vi "光源測試2.vi"() -> ()   [LabVIEW 2015]
uses:
  <vilib>/userdefined/High Color/IMAQdx.ctl
  Function/Control 5.ctl
  <vilib>/vision/Image Controls.llb/IMAQ Image.ctl
  <vilib>/vision/driver/NI_Vision_Acquisition_Software.lvlib
  <vilib>/vision/NI_Vision_Development_Module.lvlib
panel:
  in  "Action 15":bool
  in  "Action 14":bool
  in  "Action 13":bool
  in  "Action 12":bool
  in  "Action 11":bool
  out "Image 4":T1(plugin-control)
  out "error out 2":errorcluster
  out "# elements in queue":i32
  in  "Action 10":bool
  in  "Action 9":bool
  in  "Action 8(平均儲存)":bool
  in  "Action 7(キА)":bool
  in  "Action 6(清除)":bool
  out "Image 3":T1(plugin-control)
  out "Image 2":T1(plugin-control)
  out "Image 1":T1(plugin-control)
  out "Image 0":T1(plugin-control)
  out "Image":T1(plugin-control)
  out "Array":T1[](array[plugin-control])
  out "Numeric":i8 min=0 max=5 step=1
  out "Image_Array":T1[](array[typedef])
  in  "Image_Enum":T2(ring)
  in  "光源VISA":refnum<visa-resource-name>="COM14"
  out "element":T3
  in  "連續取像":bool
  in  "相機VISA":T4="cam14"
  in  "儲存影像":bool
  in  "觸發取像":bool
  in  "光源亮度 total":u8(slide) scale=0.0..255.0
  in  "milliseconds to wait":u32=200
  in  "Action 5(無)":bool
  in  "Action 4(拍照不存)":bool
  in  "Action 3(邊拍邊存)":bool
  in  "Action 2(全關)":bool
  in  "Action 1(全開)":bool
  out "回應值4":string
  out "回應值3":string
  out "回應值2":string
  out "回應值1":string
  in  "光源亮度 4":u8(slide) scale=0.0..255.0
  in  "光源亮度 3":u8(slide) scale=0.0..255.0
  in  "光源亮度 2":u8(slide) scale=0.0..255.0
  in  "光源亮度 1":u8(slide) scale=0.0..255.0
  in  "光源開啟 4":bool
  in  "光源開啟 3":bool
  in  "光源開啟 2":bool
  in  "光源開啟 1":bool
  in  "光源關閉 4":bool
  in  "光源關閉 3":bool
  in  "光源關閉 2":bool
  in  "通訊關閉":bool
  in  "光源關閉 1":bool
  in  "初始化":bool
  in  "Stop Button":bool
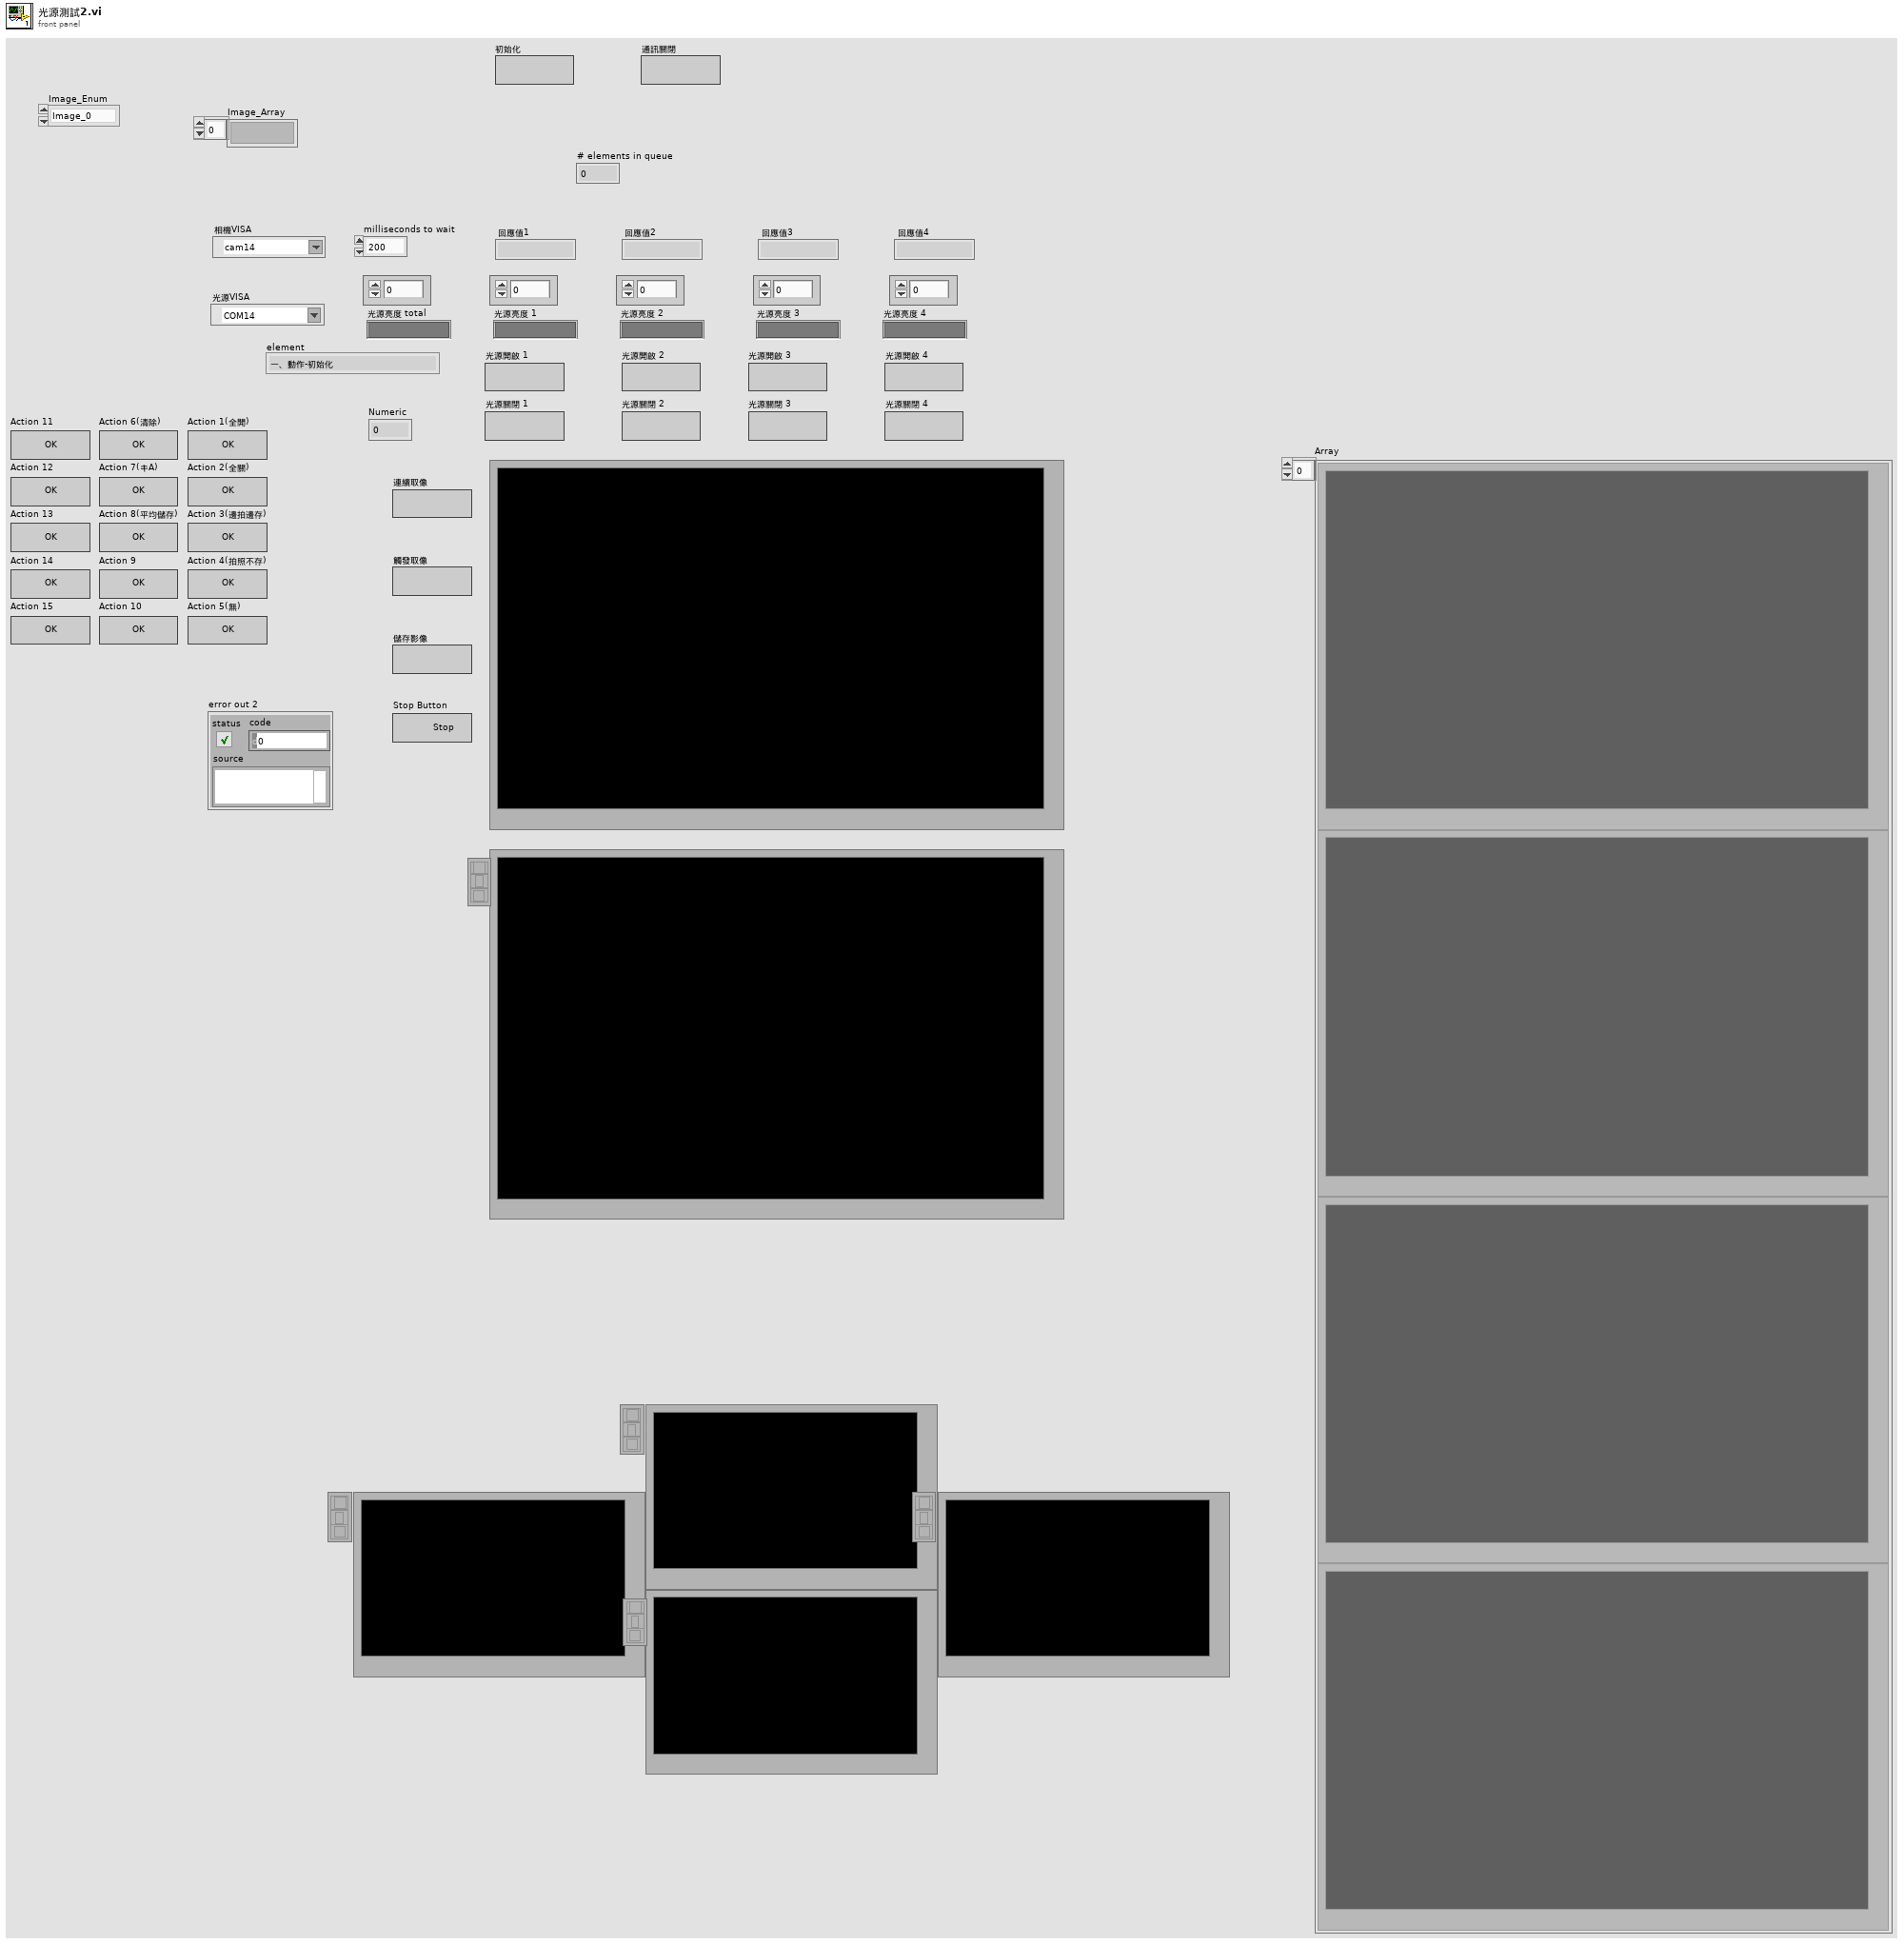
[diagram p1: front panel]
types:
  T1 = typedef "IMAQ Image.ctl" = refnum<image>
  T2 = enum16{"Image_0", "Image_1", "Image_2", "Image_3", "Image_4", "Image_5", "Image_6"}
  T3 = typedef "Control 5.ctl" = enum16{"一、動作-初始化", "二、動作-單次取像", "三、動作-連續取像", "四、動作-儲存影像", "五、動作-閒置", "六、動作-離開", "CH1_Open", "CH2_Open", "CH3_Open", "CH4_Open", "CH1_Close", "CH2_Close", "CH3_Close", "CH4_Close", "Action1", "Action2", "Action3", "Action4", "Action5", "Action6", "Action7", "Action8", "Action9", "Action10", "Action11", "Action12", "Action13", "Action14", "Action15"}
  T4 = typedef "IMAQdx.ctl" = refnum<k21>
  T5 = typedef "光源通訊_action_control.ctl" = enum16{"initial", "開啟光源", "關閉光源", "close"}
  T6 = typedef "Image Type" = u32
  T7 = typedef "LVDateTimeRec.ctl" = cluster{"fractional second":dbl, "second":i32, "minute":i32, "hour":i32, "day of month":i32, "month":i32, "year":i32, "day of week":i32, "day of year":i32, "DST":i32}
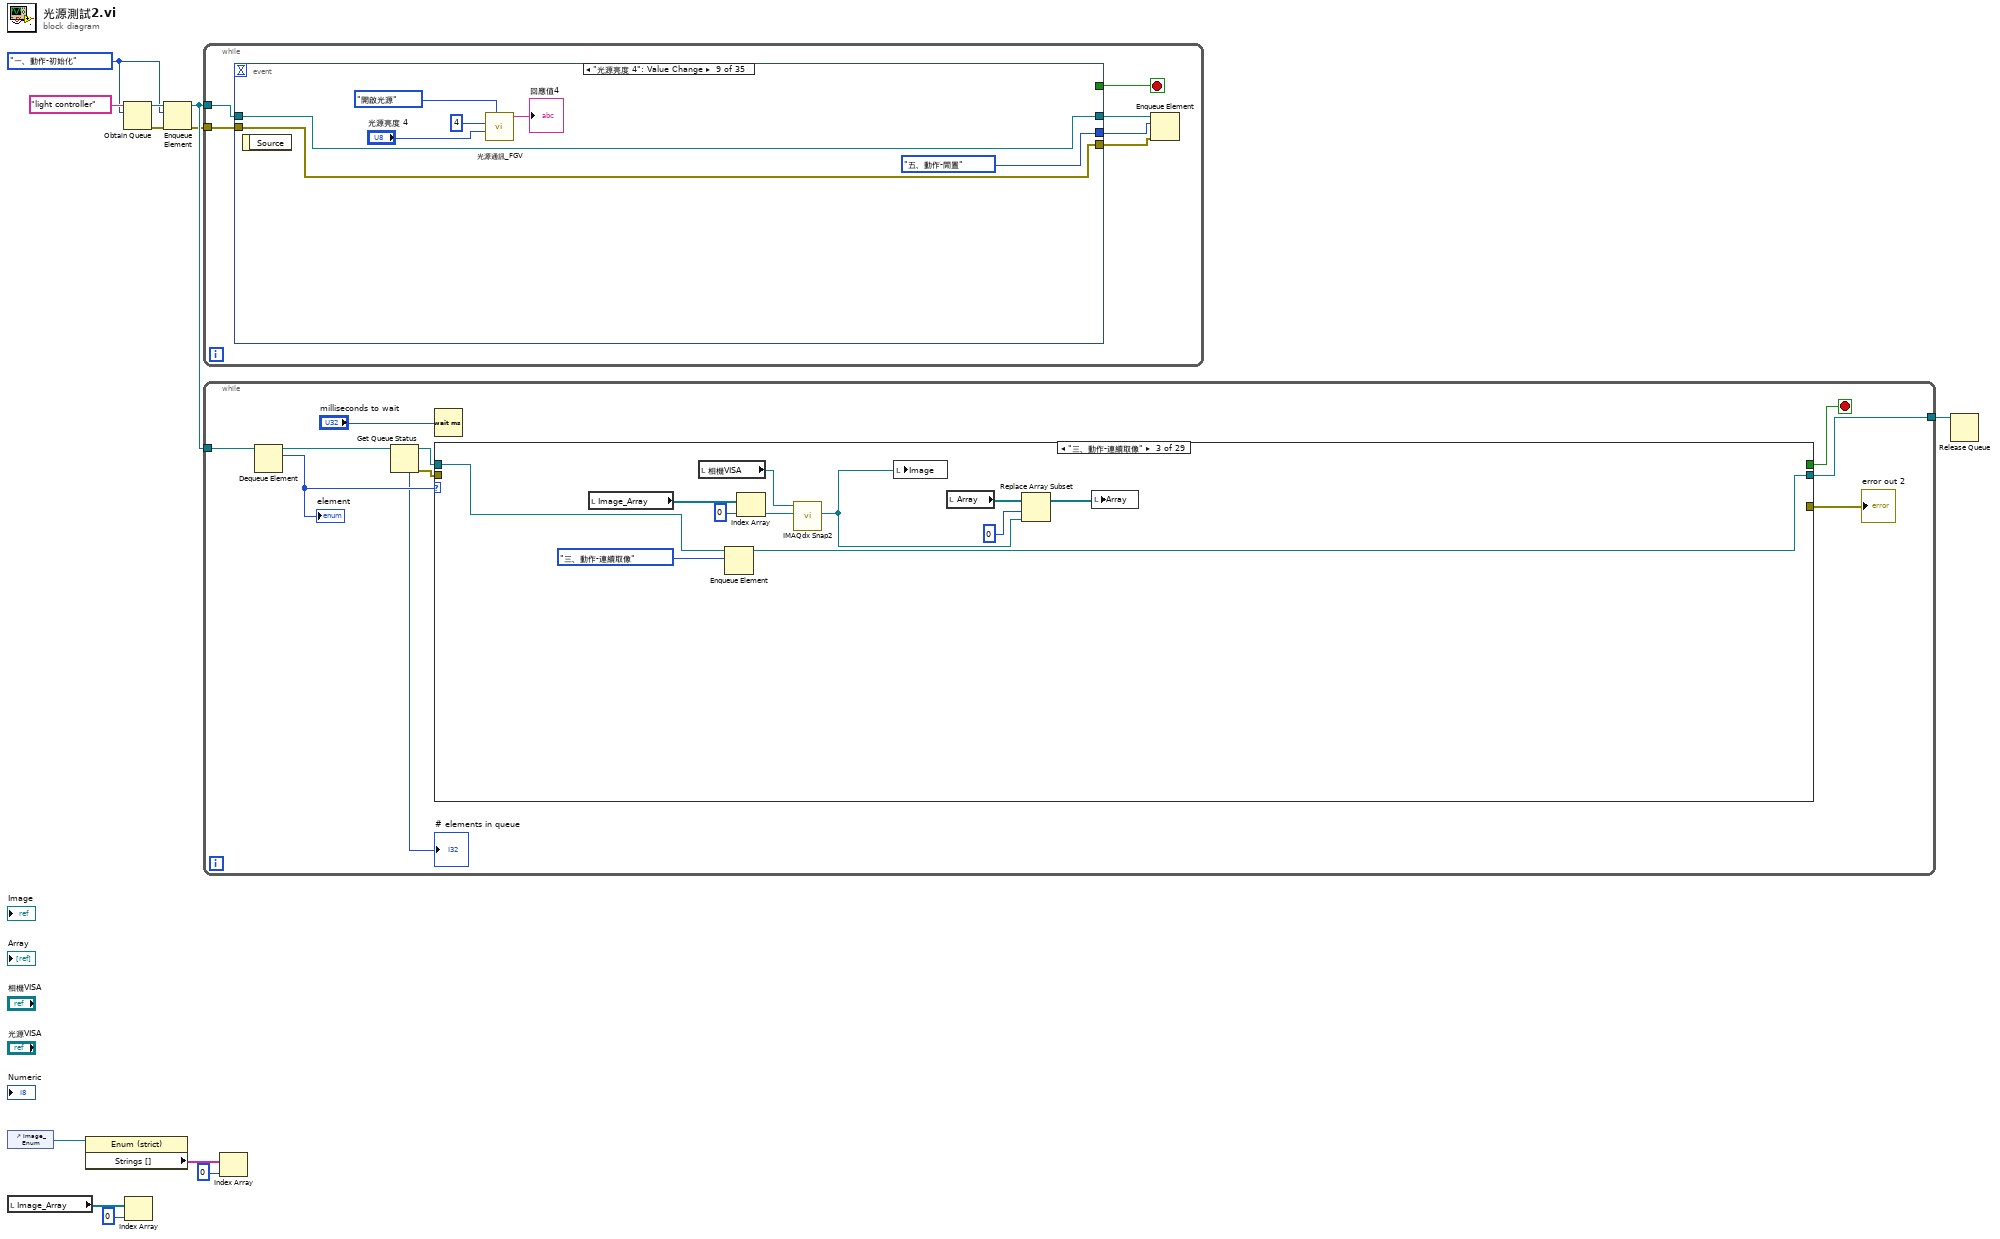
[diagram p0: block diagram]
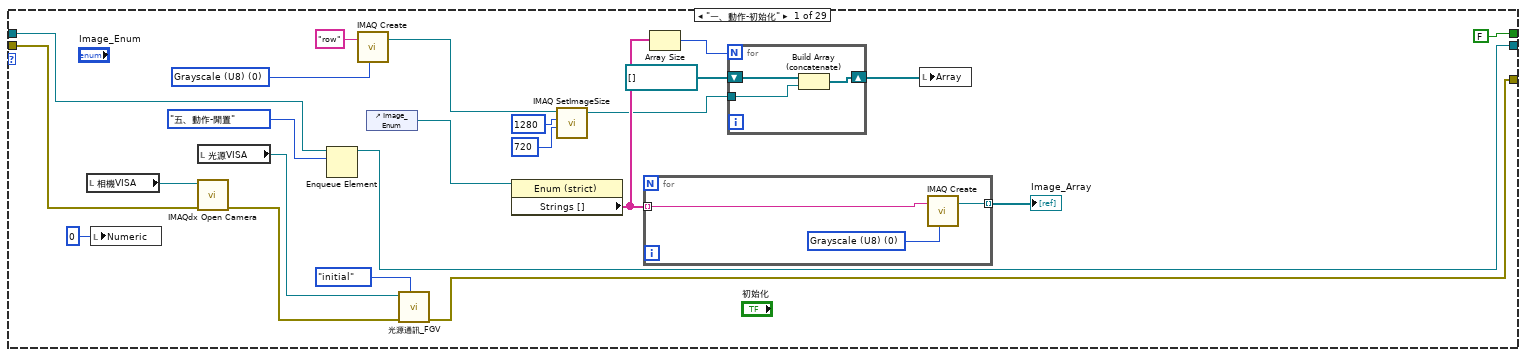
[diagram p2: hidden frame]
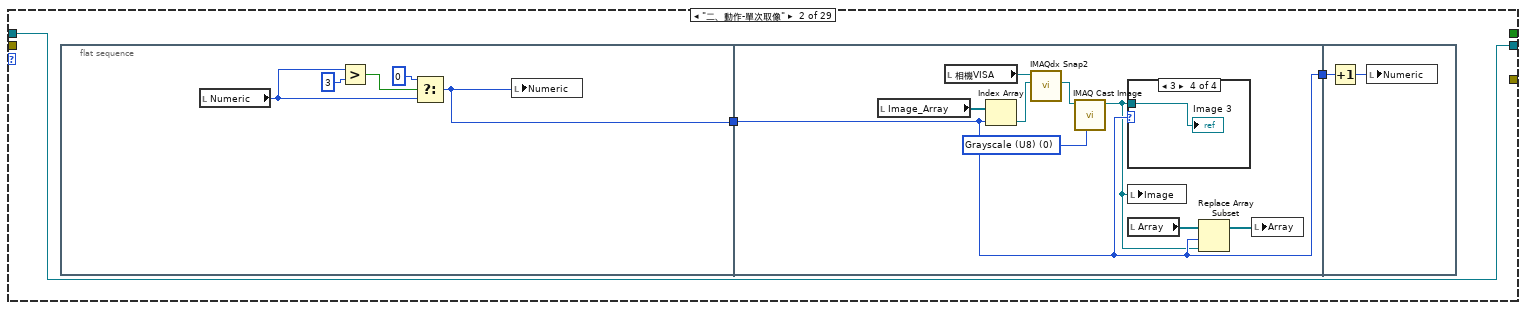
[diagram p3: hidden frame]
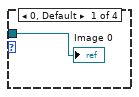
[diagram p4: hidden frame]
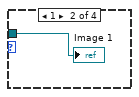
[diagram p5: hidden frame]
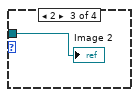
[diagram p6: hidden frame]
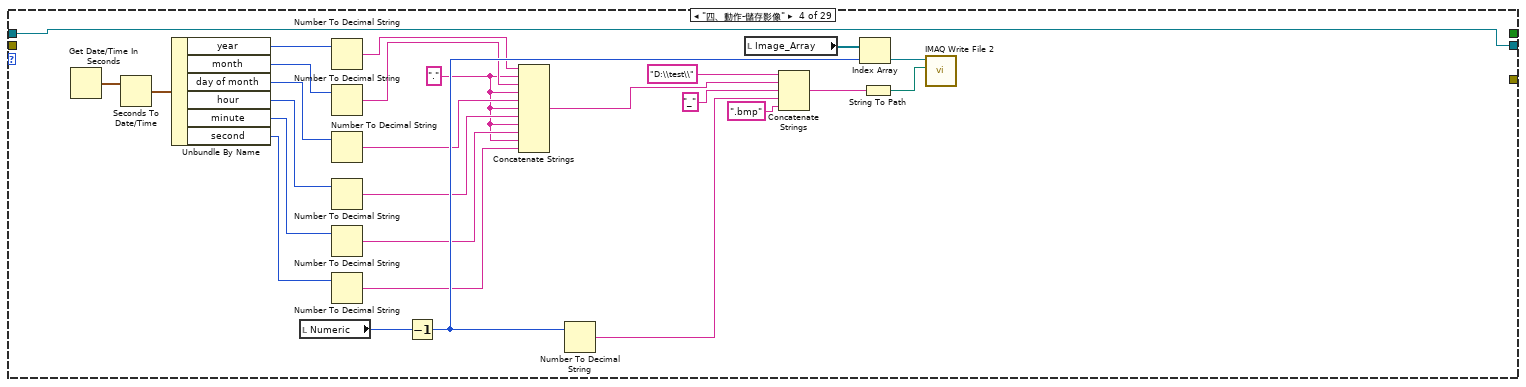
[diagram p7: hidden frame]
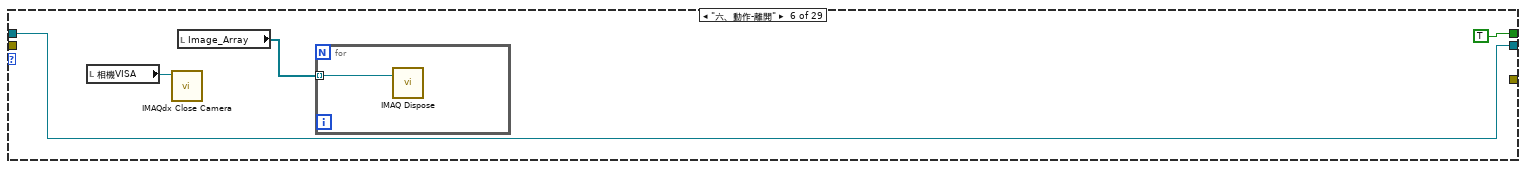
[diagram p9: hidden frame]
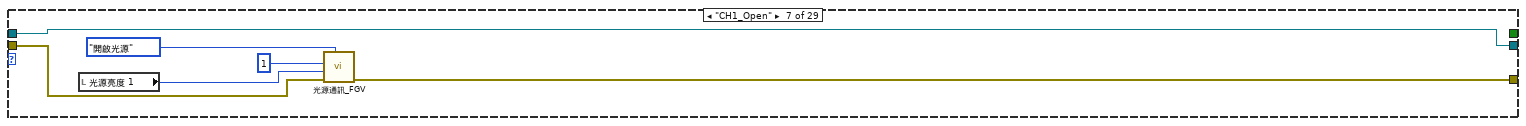
[diagram p10: hidden frame]
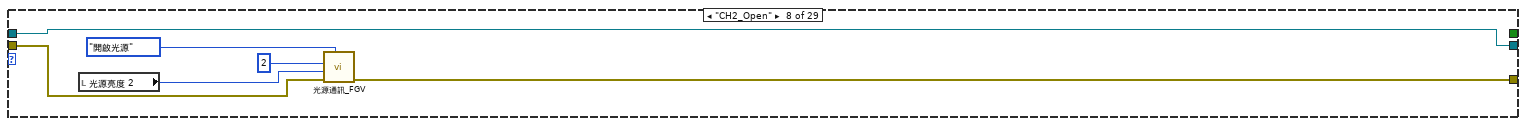
[diagram p11: hidden frame]
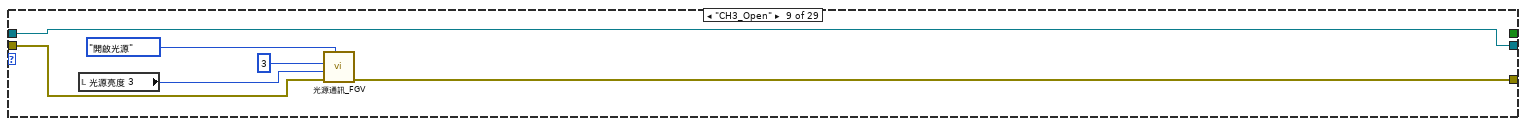
[diagram p12: hidden frame]
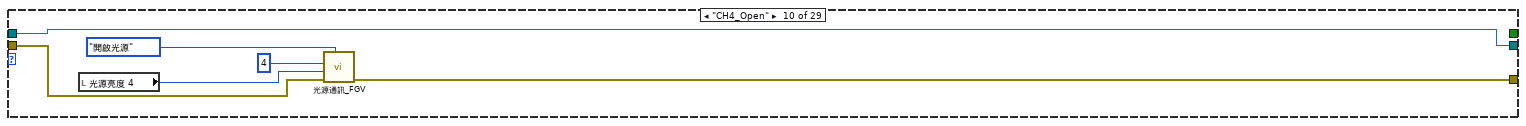
[diagram p13: hidden frame]
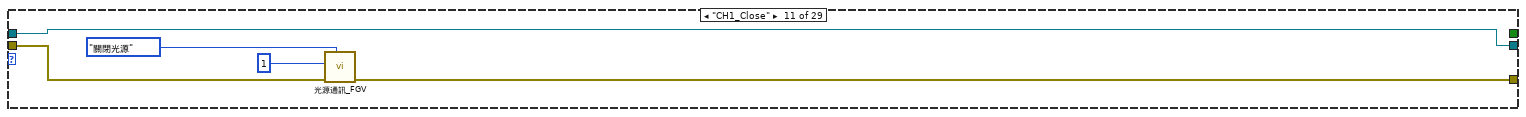
[diagram p14: hidden frame]
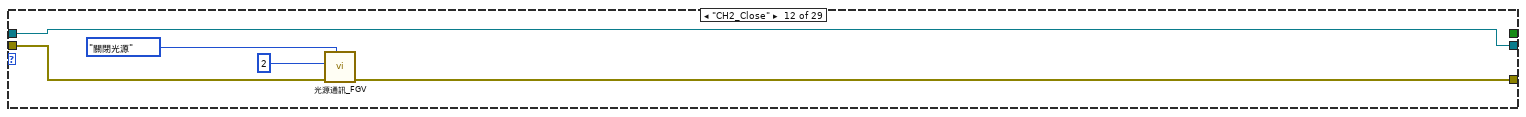
[diagram p15: hidden frame]
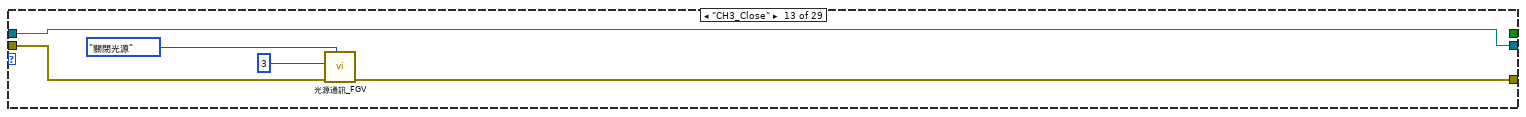
[diagram p16: hidden frame]
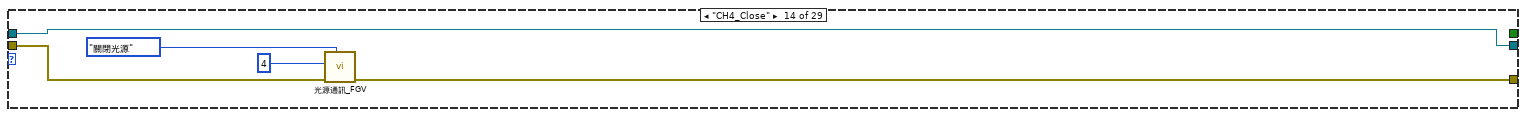
[diagram p17: hidden frame]
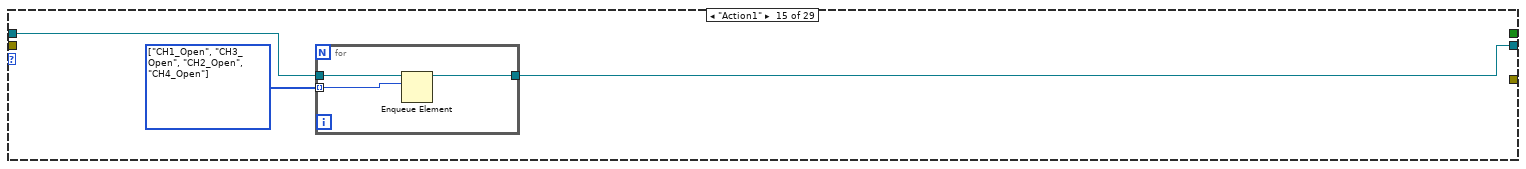
[diagram p18: hidden frame]
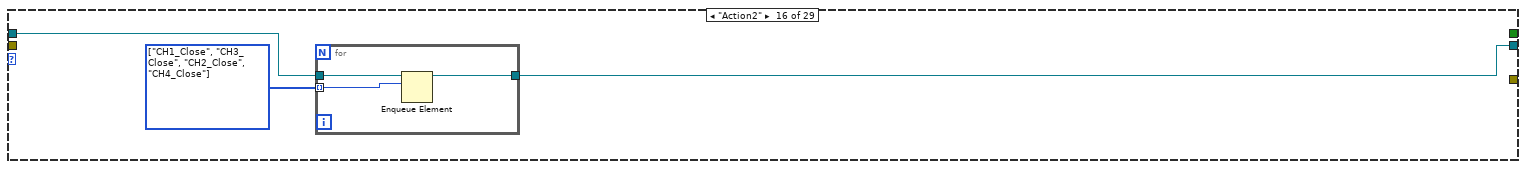
[diagram p19: hidden frame]
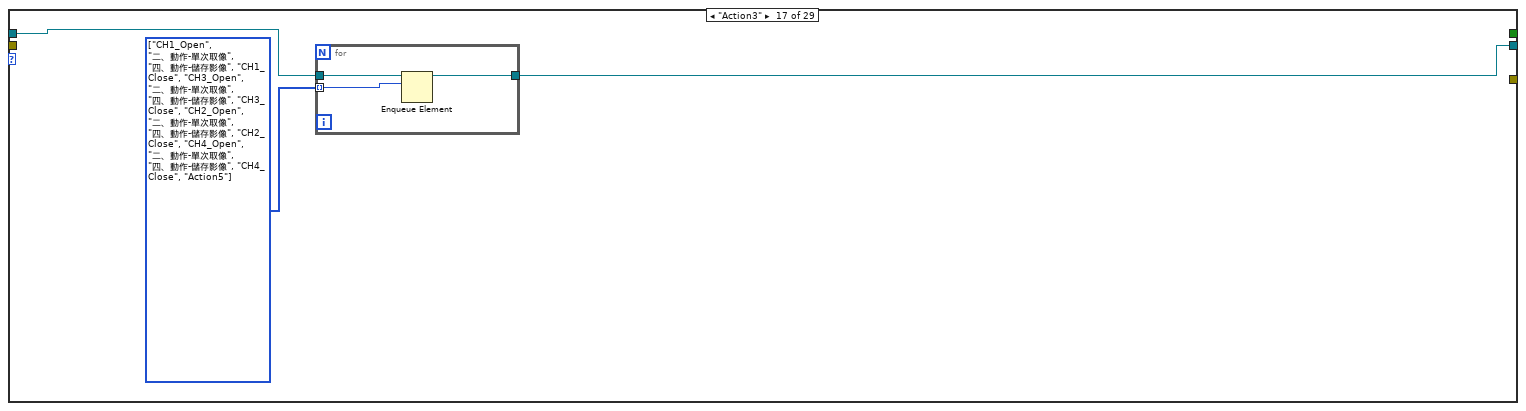
[diagram p20: hidden frame]
diagram:
  w6 = Control_5."一、動作-初始化"
  n1 = control-ref of="Image_Enum"() -> (w3:refnum<vi>)
  n2 = local read "Image_Array"() -> (w1:T1[])
  n3 = property class="Enum (strict)"(reference=w3) -> ("Strings []"=w4:string[])  [unwired: 1 in, 2 out]
  n4 = Obtain Queue(name (unnamed)="light controller", element data type=w6) -> (queue out=w10:refnum<queue>, error out=w8:errorcluster)  [unwired: 3 in, 1 out]
  n5 = Index Array(array=w1, index=0) -> ()  [unwired: 1 out]
  n6 = Enqueue Element(queue=w10, element=w6, error in (no error)=w8) -> (queue out=w9:refnum<queue>, error out=w7:errorcluster)  [unwired: 1 in, 1 out]
  n7 = while {
    tunnel: w9 -> [w17]
    tunnel: w7 -> [w13]
    stop <- w18 stop-if-true
    n8 = event shown="[8] \"光源亮度 4\": Value Change" {
      selector: _ -> [_ _ _ _ _ _ _ _ _ _ _ _ _ _ _ _ _ _ _ _ _ _ _ _ _ _ _ _ _ _ _ _ _ _ _]
      dyn-events: _ -> [_ _ _ _ _ _ _ _ _ _ _ _ _ _ _ _ _ _ _ _ _ _ _ _ _ _ _ _ _ _ _ _ _ _ _]
      timeout: _ -> [_ _ _ _ _ _ _ _ _ _ _ _ _ _ _ _ _ _ _ _ _ _ _ _ _ _ _ _ _ _ _ _ _ _ _]
      tunnel: [_ TRUE _ _ _ _ _ _ _ _ _ _ _ _ _ _ _ _ _ _ _ _ _ _ _ _ _ _ _ _ _ _ _ _ _] -> w18
      tunnel: w17 -> [w21 w24 w28 w31 w34 w37 w44 w52 w59 w66 w69 w72 w75 w78 w81 w84 w87 w89 w93 w96 w98 w103 w109 w112 w115 w118 w121 w124 w127 w130 w133 w138 w146 w148 w151]
      tunnel: [w21 w24 w28 w31 w34 w37 w44 w52 w59 w66 w69 w72 w75 w78 w81 w84 w87 w89 w93 w96 w98 w101 w109 w112 w115 w118 w121 w124 w127 w130 w133 w138 w146 w148 w151] -> w15
      tunnel: [Control_5."五、動作-閒置" Control_5."六、動作-離開" Control_5."一、動作-初始化" Control_5."CH1_Close" Control_5."五、動作-閒置" Control_5."五、動作-閒置" Control_5."五、動作-閒置" Control_5."五、動作-閒置" Control_5."五、動作-閒置" Control_5."CH2_Close" Control_5."CH3_Close" Control_5."CH4_Close" Control_5."CH1_Open" Control_5."CH2_Open" Control_5."CH3_Open" Control_5."CH4_Open" Control_5."Action1" Control_5."Action2" Control_5."Action4" Control_5."Action3" Control_5."Action5" _ Control_5."Action7" Control_5."Action8" Control_5."Action9" Control_5."Action10" Control_5."Action11" Control_5."Action12" Control_5."Action13" Control_5."Action14" Control_5."Action15" Control_5."五、動作-閒置" Control_5."二、動作-單次取像" Control_5."四、動作-儲存影像" Control_5."三、動作-連續取像"] -> w16
      tunnel: [w20 w23 w27 w30 w33 w38 w45 w51 w58 w65 w68 w71 w74 w77 w80 w83 w86 w90 w92 w95 w99 w105 w108 w111 w114 w117 w120 w123 w126 w129 w132 w137 w144 w147 w150] -> w14
      tunnel: w13 -> [w20 w23 w27 w30 w33 w38 w45 w51 w58 w65 w68 w71 w74 w77 w80 w83 w86 w90 w92 w95 w99 w105 w108 w111 w114 w117 w120 w123 w126 w129 w132 w137 w144 w147 w150]
      event Timeout {
        n9 = event-data() -> ()  [unwired: 1 in, 1 out]
      }
      event "Stop Button": Value Change {
        n10 = event-data() -> ()  [unwired: 1 in, 1 out]
      }
      event "初始化": Value Change {
        n11 = event-data() -> ()  [unwired: 1 in, 1 out]
      }
      event "光源關閉 1": Value Change {
        n12 = event-data() -> ()  [unwired: 1 in, 1 out]
      }
      event "通訊關閉": Value Change {
        n13 = event-data() -> ()  [unwired: 1 in, 1 out]
        n14 = call "光源通訊_FGV.vi"("通訊_action"=光源通訊_action_control."close") -> ()  [unwired: 9 in, 2 out]
      }
      event "光源亮度 1": Value Change {
        n15 = event-data() -> ()  [unwired: 1 in, 1 out]
        n16 = call "光源通訊_FGV.vi"("通訊_action"=光源通訊_action_control."開啟光源", "亮度"="光源亮度 1", "通道"=u8 1) -> ("回應值"=→"回應值1":string)  [unwired: 7 in, 1 out]
      }
      event "光源亮度 2": Value Change {
        n17 = event-data() -> ()  [unwired: 1 in, 1 out]
        n18 = call "光源通訊_FGV.vi"("通訊_action"=光源通訊_action_control."開啟光源", "亮度"="光源亮度 2", "通道"=u8 2) -> ("回應值"=→"回應值2":string)  [unwired: 7 in, 1 out]
      }
      event "光源亮度 3": Value Change {
        n19 = event-data() -> ()  [unwired: 1 in, 1 out]
        n20 = call "光源通訊_FGV.vi"("通訊_action"=光源通訊_action_control."開啟光源", "亮度"="光源亮度 3", "通道"=u8 3) -> ("回應值"=→"回應值3":string)  [unwired: 7 in, 1 out]
      }
      event "光源亮度 4": Value Change {
        n21 = event-data() -> ()  [unwired: 1 in, 1 out]
        n22 = call "光源通訊_FGV.vi"("通訊_action"=光源通訊_action_control."開啟光源", "亮度"="光源亮度 4", "通道"=u8 4) -> ("回應值"=→"回應值4":string)  [unwired: 7 in, 1 out]
      }
      event "光源關閉 2": Value Change {
        n23 = event-data() -> ()  [unwired: 1 in, 1 out]
      }
      event "光源關閉 3": Value Change {
        n24 = event-data() -> ()  [unwired: 1 in, 1 out]
      }
      event "光源關閉 4": Value Change {
        n25 = event-data() -> ()  [unwired: 1 in, 1 out]
      }
      event "光源開啟 1": Value Change {
        n26 = event-data() -> ()  [unwired: 1 in, 1 out]
      }
      event "光源開啟 2": Value Change {
        n27 = event-data() -> ()  [unwired: 1 in, 1 out]
      }
      event "光源開啟 3": Value Change {
        n28 = event-data() -> ()  [unwired: 1 in, 1 out]
      }
      event "光源開啟 4": Value Change {
        n29 = event-data() -> ()  [unwired: 1 in, 1 out]
      }
      event "Action 1(全開)": Value Change {
        n30 = event-data() -> ()  [unwired: 1 in, 1 out]
      }
      event "Action 2(全關)": Value Change {
        n31 = event-data() -> ()  [unwired: 1 in, 1 out]
      }
      event "Action 4(拍照不存)": Value Change {
        n32 = event-data() -> ()  [unwired: 1 in, 1 out]
      }
      event "Action 3(邊拍邊存)": Value Change {
        n33 = event-data() -> ()  [unwired: 1 in, 1 out]
      }
      event "Action 5(無)": Value Change {
        n34 = event-data() -> ()  [unwired: 1 in, 1 out]
      }
      event "Action 6(清除)": Value Change {
        n35 = event-data() -> ()  [unwired: 1 in, 1 out]
        n36 = Get Queue Status(queue=w103) -> (queue out=w100:refnum<queue>, # elements in queue=w104:i32)  [unwired: 2 in, 6 out]
        n37 = for {
          N: w104 -> [_]
          tunnel: w100 -> [w106]
          n38 = Dequeue Element(queue=w106) -> ()  [unwired: 2 in, 4 out]
        }
        n39 = Enqueue Element(queue=w100, element=Control_5."五、動作-閒置") -> (queue out=w101:refnum<queue>)  [unwired: 2 in, 2 out]
      }
      event "Action 7(キА)": Value Change {
        n40 = event-data() -> ()  [unwired: 1 in, 1 out]
      }
      event "Action 8(平均儲存)": Value Change {
        n41 = event-data() -> ()  [unwired: 1 in, 1 out]
      }
      event "Action 9": Value Change {
        n42 = event-data() -> ()  [unwired: 1 in, 1 out]
      }
      event "Action 10": Value Change {
        n43 = event-data() -> ()  [unwired: 1 in, 1 out]
      }
      event "Action 11": Value Change {
        n44 = event-data() -> ()  [unwired: 1 in, 6 out]
      }
      event "Action 12": Value Change {
        n45 = event-data() -> ()  [unwired: 1 in, 6 out]
      }
      event "Action 13": Value Change {
        n46 = event-data() -> ()  [unwired: 1 in, 6 out]
      }
      event "Action 14": Value Change {
        n47 = event-data() -> ()  [unwired: 1 in, 6 out]
      }
      event "Action 15": Value Change {
        n48 = event-data() -> ()  [unwired: 1 in, 6 out]
      }
      event "光源亮度 total": Value Change {
        n49 = event-data() -> ()  [unwired: 1 in, 1 out]
        n50 = local write "光源亮度 2"("光源亮度 total") -> ()
        n51 = local write "光源亮度 1"("光源亮度 total") -> ()
        n52 = local write "光源亮度 3"("光源亮度 total") -> ()
        n53 = local write "光源亮度 4"("光源亮度 total") -> ()
        n54 = for {
          N: 4 -> [_]
          tunnel: "光源亮度 total" -> [w140]
          tunnel: [w139] -> _ mode=indexing
          i -> [w142]
          n55 = Increment(x=w142) -> (x+1=w141:i32)
          n56 = call "光源通訊_FGV.vi"("通訊_action"=光源通訊_action_control."開啟光源", "亮度"=w140, "通道"=w141) -> ("error out"=w139:errorcluster)  [unwired: 7 in, 1 out]
        }
      }
      event "觸發取像": Value Change {
        n57 = event-data() -> ()  [unwired: 1 in, 1 out]
      }
      event "儲存影像": Value Change {
        n58 = event-data() -> ()  [unwired: 1 in, 1 out]
      }
      event "連續取像": Value Change {
        n59 = event-data() -> ()  [unwired: 1 in, 1 out]
      }
    }
    n60 = Enqueue Element(queue=w15, element=w16, error in (no error)=w14) -> ()  [unwired: 1 in, 3 out]
  }
  n61 = while {
    tunnel: [w162] -> w11
    tunnel: w9 -> [w160]
    stop <- w158 stop-if-true
    n62 = Dequeue Element(queue=w160) -> (queue out=w157:refnum<queue>, element=w159:T3)  [unwired: 2 in, 2 out]
    "element" <- w159
    n63 = Get Queue Status(queue=w157) -> (queue out=w156:refnum<queue>, error out=w154:errorcluster, # elements in queue=→"# elements in queue":i32)  [unwired: 2 in, 5 out]
    n64 = Wait (ms)(milliseconds to wait="milliseconds to wait") -> ()  [unwired: 1 out]
    n65 = case shown="\"三、動作-連續取像\"" w159 {
      tunnel: [w172 w194 w222 w249 w253 w257 w264 w270 w276 w282 w287 w292 w297 w302 w304 w310 w317 w322 w329 w335 w354 w385 w391 w397 w403 w409 w415 w421 w427] -> w162
      tunnel: w156 -> [w173 w194 w223 w249 w253 w257 w264 w270 w276 w282 w287 w292 w297 w302 w305 w311 w316 w323 w330 w334 w355 w386 w392 w398 w404 w410 w416 w422 w428]
      tunnel: [FALSE _ _ _ _ TRUE _ _ _ _ _ _ _ _ _ _ _ _ _ _ _ _ _ _ _ _ _ _ _] -> w158
      tunnel: w154 -> [w170 _ _ _ _ _ w260 w266 w272 w278 w284 w289 w294 w299 _ _ _ _ _ _ _ _ _ _ _ _ _ _ _]
      tunnel: [w171 _ _ _ _ _ w259 w265 w271 w277 w283 w288 w293 w298 _ _ _ _ _ _ _ _ _ _ _ _ _ _ _] -> w153
      frame "一、動作-初始化" {
        w163 = T6 0 items=["Grayscale (U8)", "Grayscale (I16)", "Grayscale (SGL)", "Complex (CSG)", "RGB (U32)", "HSL (U32)", "RGB (U64)", "Grayscale (U16)"] ("Image Type")
        n66 = local read "相機VISA"() -> (w183:T4)
        n67 = local write "Numeric"(i8 0 ("Numeric")) -> ()
        n68 = local read "光源VISA"() -> (w180:refnum<visa-resource-name>)
        n69 = call <vilib>:"IMAQdx Open Camera.vi"("error in"=w170, "Session In"=w183) -> ("error out"=w169:errorcluster)  [unwired: 8 in, 1 out]
        n70 = Enqueue Element(queue=w173, element=Control_5."五、動作-閒置") -> (queue out=w172:refnum<queue>)  [unwired: 2 in, 2 out]
        n71 = call "IMAQ Create"("Image Name"="row", "Image Type"=w163) -> ("New Image"=w178:T1)  [unwired: 3 in, 1 out]
        n72 = control-ref of="Image_Enum"() -> (w182:refnum<vi>)
        n73 = call "光源通訊_FGV.vi"("通訊_action"=光源通訊_action_control."initial", "error in (no error)"=w169, "VISA resource name"=w180) -> ("error out"=w171:errorcluster)  [unwired: 7 in, 1 out]
        n74 = property class="Enum (strict)"(reference=w182) -> ("Strings []"=w168:string[])  [unwired: 1 in, 2 out]
        n75 = call "IMAQ SetImageSize"("Y Resolution"=720, "X Resolution"=1280, "Image"=w178) -> ("Image Out"=w166:T1)  [unwired: 2 in, 1 out]
        n76 = for {
          tunnel: w168 -> [w191] mode=indexing
          tunnel: [w189] -> w181 mode=indexing
          w190 = T6 0 items=["Grayscale (U8)", "Grayscale (I16)", "Grayscale (SGL)", "Complex (CSG)", "RGB (U32)", "HSL (U32)", "RGB (U64)", "Grayscale (U16)"] ("Image Type")
          n77 = call "IMAQ Create"("Image Name"=w191, "Image Type"=w190) -> ("New Image"=w189:T1)  [unwired: 3 in, 1 out]
        }
        "Image_Array" <- w181
        n78 = Array Size(array=w168) -> (size(s)=w167:i32)
        n79 = for {
          N: w167 -> [_]
          tunnel: w166 -> [w187]
          shift-right: [w188] -> w164
          shift-left: T1[] [] -> [w186]
          n80 = Build Array (concatenate)(w186, w187) -> (w188:T1[])
        }
        n81 = local write "Array"(w164) -> ()
      }
      frame "二、動作-單次取像" {
        n82 = flat-sequence {
          tunnel: [w195] -> w193
          tunnel: w193 -> [w203]
          tunnel: [w203] -> w192
          tunnel: w192 -> [w213]
          frame #0 {
            n83 = local read "Numeric"() -> (w199:i8)
            n84 = Greater?(x=w199, y=i8 3) -> (0:w197:bool)
            n85 = Select(t=i8 0 ("y"), s=w197, f=w199) -> (s? t:f=w195:i8)
            n86 = local write "Numeric"(w195) -> ()
          }
          frame #1 {
            w202 = T6 0 items=["Grayscale (U8)", "Grayscale (I16)", "Grayscale (SGL)", "Complex (CSG)", "RGB (U32)", "HSL (U32)", "RGB (U64)", "Grayscale (U16)"] ("Image Type")
            n87 = local read "Image_Array"() -> (w206:T1[])
            n88 = local read "相機VISA"() -> (w208:T4)
            n89 = Index Array(array=w206, index=w203) -> (element=w207:T1)
            n90 = call <vilib>:"IMAQdx Snap2.vi"("Image In"=w207, "Session In"=w208) -> ("Image Out"=w201:T1)  [unwired: 7 in, 2 out]
            n91 = call "IMAQ Cast Image"("Image Type"=w202, "Image Src"=w201) -> ("Image Dst Out"=w200:T1)  [unwired: 8 in, 1 out]
            n92 = case shown="3" w203 {
              tunnel: w200 -> [w209 w210 w211 w212]
              frame 0, Default {
                "Image 0" <- w209
              }
              frame 1 {
                "Image 1" <- w210
              }
              frame 2 {
                "Image 2" <- w211
              }
              frame 3 {
                "Image 3" <- w212
              }
            }
            n93 = local write "Image"(w200) -> ()
            n94 = local read "Array"() -> (w205:T1[])
            n95 = Replace Array Subset(array=w205, new element=w200, index=w203) -> (w204:T1[])
            n96 = local write "Array"(w204) -> ()
          }
          frame #2 {
            n97 = Increment(x=w213) -> (x+1=w214:i8)
            n98 = local write "Numeric"(w214) -> ()
          }
        }
      }
      frame "三、動作-連續取像" {
        n99 = local read "Image_Array"() -> (w221:T1[])
        n100 = local read "相機VISA"() -> (w225:T4)
        n101 = Enqueue Element(queue=w223, element=Control_5."三、動作-連續取像") -> (queue out=w222:refnum<queue>)  [unwired: 2 in, 2 out]
        n102 = Index Array(array=w221, index=0) -> (element=w219:T1)
        n103 = call <vilib>:"IMAQdx Snap2.vi"("Image In"=w219, "Session In"=w225) -> ("Image Out"=w215:T1)  [unwired: 7 in, 2 out]
        n104 = local write "Image"(w215) -> ()
        n105 = local read "Array"() -> (w217:T1[])
        n106 = Replace Array Subset(array=w217, new element=w215, index=0) -> (w216:T1[])
        n107 = local write "Array"(w216) -> ()
      }
      frame "四、動作-儲存影像" {
        w227 = "."
        n108 = Get Date/Time In Seconds() -> (seconds since 1Jan1904=w248:timestamp)
        n109 = Seconds To Date/Time(time stamp (now)=w248) -> (date time rec=w247:T7)  [unwired: 1 in]
        n110 = Unbundle By Name(w247) -> ("year"=w246:i32, "month"=w245:i32, "day of month"=w244:i32, "hour"=w243:i32, "minute"=w242:i32, "second"=w241:i32)
        n111 = local read "Numeric"() -> (w238:i8)
        n112 = Number To Decimal String(number=w246) -> (decimal integer string=w233:string)  [unwired: 1 in]
        n113 = Number To Decimal String(number=w245) -> (decimal integer string=w232:string)  [unwired: 1 in]
        n114 = Number To Decimal String(number=w244) -> (decimal integer string=w231:string)  [unwired: 1 in]
        n115 = Number To Decimal String(number=w243) -> (decimal integer string=w230:string)  [unwired: 1 in]
        n116 = Number To Decimal String(number=w242) -> (decimal integer string=w229:string)  [unwired: 1 in]
        n117 = Number To Decimal String(number=w241) -> (decimal integer string=w228:string)  [unwired: 1 in]
        n118 = Decrement(x=w238) -> (x-1=w234:i8)
        n119 = Concatenate Strings(w233, w227, w232, w227, w231, w227, w230, w227, w229, w227, w228) -> (w226:string)
        n120 = Number To Decimal String(number=w234) -> (decimal integer string=w235:string)  [unwired: 1 in]
        n121 = local read "Image_Array"() -> (w240:T1[])
        n122 = Concatenate Strings("D:\\test\\" ("string"), w226, "_" ("string"), w235, ".bmp" ("string")) -> (w251:string)
        n123 = Index Array(array=w240, index=w234) -> (element=w239:T1)
        n124 = String To Path(string=w251) -> (path=w250:path)
        n125 = call-poly "IMAQ Write File 2"("File Path"=w250, "Image"=w239) -> ()  [unwired: 8 in, 2 out]
      }
      frame "五、動作-閒置", Default {
      }
      frame "六、動作-離開" {
        n126 = local read "相機VISA"() -> (w255:T4)
        n127 = call <vilib>:"IMAQdx Close Camera.vi"("Session In"=w255) -> ()  [unwired: 10 in, 1 out]
        n128 = local read "Image_Array"() -> (w254:T1[])
        n129 = for {
          tunnel: w254 -> [w258] mode=indexing
          n130 = call "IMAQ Dispose"("Image"=w258) -> ()  [unwired: 5 in, 1 out]
        }
      }
      frame "CH1_Open" {
        n131 = local read "光源亮度 1"() -> (w263:u8)
        n132 = call "光源通訊_FGV.vi"("通訊_action"=光源通訊_action_control."開啟光源", "error in (no error)"=w260, "亮度"=w263, "通道"=u8 1) -> ("error out"=w259:errorcluster)  [unwired: 6 in, 1 out]
      }
      frame "CH2_Open" {
        n133 = local read "光源亮度 2"() -> (w269:u8)
        n134 = call "光源通訊_FGV.vi"("通訊_action"=光源通訊_action_control."開啟光源", "error in (no error)"=w266, "亮度"=w269, "通道"=u8 2) -> ("error out"=w265:errorcluster)  [unwired: 6 in, 1 out]
      }
      frame "CH3_Open" {
        n135 = local read "光源亮度 3"() -> (w275:u8)
        n136 = call "光源通訊_FGV.vi"("通訊_action"=光源通訊_action_control."開啟光源", "error in (no error)"=w272, "亮度"=w275, "通道"=u8 3) -> ("error out"=w271:errorcluster)  [unwired: 6 in, 1 out]
      }
      frame "CH4_Open" {
        n137 = local read "光源亮度 4"() -> (w281:u8)
        n138 = call "光源通訊_FGV.vi"("通訊_action"=光源通訊_action_control."開啟光源", "error in (no error)"=w278, "亮度"=w281, "通道"=u8 4) -> ("error out"=w277:errorcluster)  [unwired: 6 in, 1 out]
      }
      frame "CH1_Close" {
        n139 = call "光源通訊_FGV.vi"("通訊_action"=光源通訊_action_control."關閉光源", "error in (no error)"=w284, "通道"=u8 1) -> ("error out"=w283:errorcluster)  [unwired: 7 in, 1 out]
      }
      frame "CH2_Close" {
        n140 = call "光源通訊_FGV.vi"("通訊_action"=光源通訊_action_control."關閉光源", "error in (no error)"=w289, "通道"=u8 2) -> ("error out"=w288:errorcluster)  [unwired: 7 in, 1 out]
      }
      frame "CH3_Close" {
        n141 = call "光源通訊_FGV.vi"("通訊_action"=光源通訊_action_control."關閉光源", "error in (no error)"=w294, "通道"=u8 3) -> ("error out"=w293:errorcluster)  [unwired: 7 in, 1 out]
      }
      frame "CH4_Close" {
        n142 = call "光源通訊_FGV.vi"("通訊_action"=光源通訊_action_control."關閉光源", "error in (no error)"=w299, "通道"=u8 4) -> ("error out"=w298:errorcluster)  [unwired: 7 in, 1 out]
      }
      frame "Action1" {
        w303 = T3[] [enum."CH1_Open", enum."CH3_Open", enum."CH2_Open", enum."CH4_Open"] items=["一、動作-初始化", "二、動作-單次取像", "三、動作-連續取像", "四、動作-儲存影像", "五、動作-閒置", "六、動作-離開", "CH1_Open", "CH2_Open", "CH3_Open", "CH4_Open", "CH1_Close", "CH2_Close", "CH3_Close", "CH4_Close", "Action1", "Action2", "Action3", "Action4", "Action5", "Action6", "Action7", "Action8", "Action9", "Action10", "Action11", "Action12", "Action13", "Action14", "Action15"]
        n143 = for {
          tunnel: w305 -> [w308]
          tunnel: [w307] -> w304
          tunnel: w303 -> [w306] mode=indexing
          n144 = Enqueue Element(queue=w308, element=w306) -> (queue out=w307:refnum<queue>)  [unwired: 2 in, 2 out]
        }
      }
      frame "Action2" {
        w309 = T3[] [enum."CH1_Close", enum."CH3_Close", enum."CH2_Close", enum."CH4_Close"] items=["一、動作-初始化", "二、動作-單次取像", "三、動作-連續取像", "四、動作-儲存影像", "五、動作-閒置", "六、動作-離開", "CH1_Open", "CH2_Open", "CH3_Open", "CH4_Open", "CH1_Close", "CH2_Close", "CH3_Close", "CH4_Close", "Action1", "Action2", "Action3", "Action4", "Action5", "Action6", "Action7", "Action8", "Action9", "Action10", "Action11", "Action12", "Action13", "Action14", "Action15"]
        n145 = for {
          tunnel: w311 -> [w314]
          tunnel: [w313] -> w310
          tunnel: w309 -> [w312] mode=indexing
          n146 = Enqueue Element(queue=w314, element=w312) -> (queue out=w313:refnum<queue>)  [unwired: 2 in, 2 out]
        }
      }
      frame "Action3" {
        w315 = T3[] [enum."CH1_Open", enum."二、動作-單次取像", enum."四、動作-儲存影像", enum."CH1_Close", enum."CH3_Open", enum."二、動作-單次取像", enum."四、動作-儲存影像", enum."CH3_Close", enum."CH2_Open", enum."二、動作-單次取像", enum."四、動作-儲存影像", enum."CH2_Close", enum."CH4_Open", enum."二、動作-單次取像", enum."四、動作-儲存影像", enum."CH4_Close", enum."Action5"] items=["一、動作-初始化", "二、動作-單次取像", "三、動作-連續取像", "四、動作-儲存影像", "五、動作-閒置", "六、動作-離開", "CH1_Open", "CH2_Open", "CH3_Open", "CH4_Open", "CH1_Close", "CH2_Close", "CH3_Close", "CH4_Close", "Action1", "Action2", "Action3", "Action4", "Action5", "Action6", "Action7", "Action8", "Action9", "Action10", "Action11", "Action12", "Action13", "Action14", "Action15"]
        n147 = for {
          tunnel: w316 -> [w320]
          tunnel: [w319] -> w317
          tunnel: w315 -> [w318] mode=indexing
          n148 = Enqueue Element(queue=w320, element=w318) -> (queue out=w319:refnum<queue>)  [unwired: 2 in, 2 out]
        }
      }
      frame "Action4" {
        w321 = T3[] [enum."CH1_Open", enum."二、動作-單次取像", enum."CH1_Close", enum."CH3_Open", enum."二、動作-單次取像", enum."CH3_Close", enum."CH2_Open", enum."二、動作-單次取像", enum."CH2_Close", enum."CH4_Open", enum."二、動作-單次取像", enum."CH4_Close", enum."Action5"] items=["一、動作-初始化", "二、動作-單次取像", "三、動作-連續取像", "四、動作-儲存影像", "五、動作-閒置", "六、動作-離開", "CH1_Open", "CH2_Open", "CH3_Open", "CH4_Open", "CH1_Close", "CH2_Close", "CH3_Close", "CH4_Close", "Action1", "Action2", "Action3", "Action4", "Action5", "Action6", "Action7", "Action8", "Action9", "Action10", "Action11", "Action12", "Action13", "Action14", "Action15"]
        n149 = for {
          tunnel: w323 -> [w326]
          tunnel: [w325] -> w322
          tunnel: w321 -> [w324] mode=indexing
          n150 = Enqueue Element(queue=w326, element=w324) -> (queue out=w325:refnum<queue>)  [unwired: 2 in, 2 out]
        }
      }
      frame "Action5" {
        w328 = T3[] [enum."五、動作-閒置"] items=["一、動作-初始化", "二、動作-單次取像", "三、動作-連續取像", "四、動作-儲存影像", "五、動作-閒置", "六、動作-離開", "CH1_Open", "CH2_Open", "CH3_Open", "CH4_Open", "CH1_Close", "CH2_Close", "CH3_Close", "CH4_Close", "Action1", "Action2", "Action3", "Action4", "Action5", "Action6", "Action7", "Action8", "Action9", "Action10", "Action11", "Action12", "Action13", "Action14", "Action15"]
        n151 = local write "Numeric"(0) -> ()
        n152 = for {
          tunnel: w330 -> [w333]
          tunnel: [w332] -> w329
          tunnel: w328 -> [w331] mode=indexing
          n153 = Enqueue Element(queue=w333, element=w331) -> (queue out=w332:refnum<queue>)  [unwired: 2 in, 2 out]
        }
      }
      frame "Action6" {
        w336 = T3[] [enum."五、動作-閒置"] items=["一、動作-初始化", "二、動作-單次取像", "三、動作-連續取像", "四、動作-儲存影像", "五、動作-閒置", "六、動作-離開", "CH1_Open", "CH2_Open", "CH3_Open", "CH4_Open", "CH1_Close", "CH2_Close", "CH3_Close", "CH4_Close", "Action1", "Action2", "Action3", "Action4", "Action5", "Action6", "Action7", "Action8", "Action9", "Action10", "Action11", "Action12", "Action13", "Action14", "Action15"]
        n154 = for {
          tunnel: w334 -> [w339]
          tunnel: [w338] -> w335
          tunnel: w336 -> [w337] mode=indexing
          n155 = Enqueue Element(queue=w339, element=w337) -> (queue out=w338:refnum<queue>)  [unwired: 2 in, 2 out]
        }
      }
      frame "Action7" {
        w356 = T3[] [enum."五、動作-閒置"] items=["一、動作-初始化", "二、動作-單次取像", "三、動作-連續取像", "四、動作-儲存影像", "五、動作-閒置", "六、動作-離開", "CH1_Open", "CH2_Open", "CH3_Open", "CH4_Open", "CH1_Close", "CH2_Close", "CH3_Close", "CH4_Close", "Action1", "Action2", "Action3", "Action4", "Action5", "Action6", "Action7", "Action8", "Action9", "Action10", "Action11", "Action12", "Action13", "Action14", "Action15"]
        n156 = local read "Image_Array"() -> (w351:T1[])
        n157 = local read "Image_Array"() -> (w352:T1[])
        n158 = Index Array(array=w351, index #1=0, index #2=1, index #3=2, index #4=3) -> (element #1=w346:T1, element #2=w345:T1, element #3=w344:T1, element #4=w343:T1)
        n159 = for {
          tunnel: w355 -> [w359]
          tunnel: [w358] -> w354
          tunnel: w356 -> [w357] mode=indexing
          n160 = Enqueue Element(queue=w359, element=w357) -> (queue out=w358:refnum<queue>)  [unwired: 2 in, 2 out]
        }
        n161 = Build Array(w346, w345, w344, w343) -> (w342:T1[])
        n162 = Index Array(array=w352, index=4) -> (element=w341:T1)
        n163 = call "IMAQ Compute Average Image"("Image Dst"=w341, "Images"=w342) -> ("Image Dst Out"=→"Image 4":T1)  [unwired: 8 in, 1 out]
      }
      frame "Action8" {
        w364 = "."
        w387 = T3[] [enum."五、動作-閒置"] items=["一、動作-初始化", "二、動作-單次取像", "三、動作-連續取像", "四、動作-儲存影像", "五、動作-閒置", "六、動作-離開", "CH1_Open", "CH2_Open", "CH3_Open", "CH4_Open", "CH1_Close", "CH2_Close", "CH3_Close", "CH4_Close", "Action1", "Action2", "Action3", "Action4", "Action5", "Action6", "Action7", "Action8", "Action9", "Action10", "Action11", "Action12", "Action13", "Action14", "Action15"]
        n164 = Get Date/Time In Seconds() -> (seconds since 1Jan1904=w381:timestamp)
        n165 = Seconds To Date/Time(time stamp (now)=w381) -> (date time rec=w380:T7)  [unwired: 1 in]
        n166 = Unbundle By Name(w380) -> ("year"=w379:i32, "month"=w378:i32, "day of month"=w377:i32, "hour"=w376:i32, "minute"=w375:i32, "second"=w374:i32)
        n167 = Number To Decimal String(number=w379) -> (decimal integer string=w370:string)  [unwired: 1 in]
        n168 = Number To Decimal String(number=w378) -> (decimal integer string=w369:string)  [unwired: 1 in]
        n169 = Number To Decimal String(number=w377) -> (decimal integer string=w368:string)  [unwired: 1 in]
        n170 = Number To Decimal String(number=w376) -> (decimal integer string=w367:string)  [unwired: 1 in]
        n171 = Number To Decimal String(number=w375) -> (decimal integer string=w366:string)  [unwired: 1 in]
        n172 = Number To Decimal String(number=w374) -> (decimal integer string=w365:string)  [unwired: 1 in]
        n173 = for {
          tunnel: w386 -> [w390]
          tunnel: [w389] -> w385
          tunnel: w387 -> [w388] mode=indexing
          n174 = Enqueue Element(queue=w390, element=w388) -> (queue out=w389:refnum<queue>)  [unwired: 2 in, 2 out]
        }
        n175 = Concatenate Strings(w370, w364, w369, w364, w368, w364, w367, w364, w366, w364, w365) -> (w363:string)
        n176 = local read "Image_Array"() -> (w362:T1[])
        n177 = Concatenate Strings("D:\\test\\" ("string"), w363, "_" ("string"), "Ave" ("string"), ".bmp" ("string")) -> (w383:string)
        n178 = String To Path(string=w383) -> (path=w382:path)
        n179 = Index Array(array=w362, index=4) -> (element=w373:T1)
        n180 = call-poly "IMAQ Write File 2"("File Path"=w382, "Image"=w373) -> ()  [unwired: 8 in, 2 out]
      }
      frame "Action9" {
        w393 = T3[] [enum."五、動作-閒置"] items=["一、動作-初始化", "二、動作-單次取像", "三、動作-連續取像", "四、動作-儲存影像", "五、動作-閒置", "六、動作-離開", "CH1_Open", "CH2_Open", "CH3_Open", "CH4_Open", "CH1_Close", "CH2_Close", "CH3_Close", "CH4_Close", "Action1", "Action2", "Action3", "Action4", "Action5", "Action6", "Action7", "Action8", "Action9", "Action10", "Action11", "Action12", "Action13", "Action14", "Action15"]
        n181 = for {
          tunnel: w392 -> [w396]
          tunnel: [w395] -> w391
          tunnel: w393 -> [w394] mode=indexing
          n182 = Enqueue Element(queue=w396, element=w394) -> (queue out=w395:refnum<queue>)  [unwired: 2 in, 2 out]
        }
      }
      frame "Action10" {
        w399 = T3[] [enum."五、動作-閒置"] items=["一、動作-初始化", "二、動作-單次取像", "三、動作-連續取像", "四、動作-儲存影像", "五、動作-閒置", "六、動作-離開", "CH1_Open", "CH2_Open", "CH3_Open", "CH4_Open", "CH1_Close", "CH2_Close", "CH3_Close", "CH4_Close", "Action1", "Action2", "Action3", "Action4", "Action5", "Action6", "Action7", "Action8", "Action9", "Action10", "Action11", "Action12", "Action13", "Action14", "Action15"]
        n183 = for {
          tunnel: w398 -> [w402]
          tunnel: [w401] -> w397
          tunnel: w399 -> [w400] mode=indexing
          n184 = Enqueue Element(queue=w402, element=w400) -> (queue out=w401:refnum<queue>)  [unwired: 2 in, 2 out]
        }
      }
      frame "Action11" {
        w405 = T3[] [enum."五、動作-閒置"] items=["一、動作-初始化", "二、動作-單次取像", "三、動作-連續取像", "四、動作-儲存影像", "五、動作-閒置", "六、動作-離開", "CH1_Open", "CH2_Open", "CH3_Open", "CH4_Open", "CH1_Close", "CH2_Close", "CH3_Close", "CH4_Close", "Action1", "Action2", "Action3", "Action4", "Action5", "Action6", "Action7", "Action8", "Action9", "Action10", "Action11", "Action12", "Action13", "Action14", "Action15"]
        n185 = for {
          tunnel: w404 -> [w408]
          tunnel: [w407] -> w403
          tunnel: w405 -> [w406] mode=indexing
          n186 = Enqueue Element(queue=w408, element=w406) -> (queue out=w407:refnum<queue>)  [unwired: 2 in, 2 out]
        }
      }
      frame "Action12" {
        w411 = T3[] [enum."五、動作-閒置"] items=["一、動作-初始化", "二、動作-單次取像", "三、動作-連續取像", "四、動作-儲存影像", "五、動作-閒置", "六、動作-離開", "CH1_Open", "CH2_Open", "CH3_Open", "CH4_Open", "CH1_Close", "CH2_Close", "CH3_Close", "CH4_Close", "Action1", "Action2", "Action3", "Action4", "Action5", "Action6", "Action7", "Action8", "Action9", "Action10", "Action11", "Action12", "Action13", "Action14", "Action15"]
        n187 = for {
          tunnel: w410 -> [w414]
          tunnel: [w413] -> w409
          tunnel: w411 -> [w412] mode=indexing
          n188 = Enqueue Element(queue=w414, element=w412) -> (queue out=w413:refnum<queue>)  [unwired: 2 in, 2 out]
        }
      }
      frame "Action13" {
        w417 = T3[] [enum."五、動作-閒置"] items=["一、動作-初始化", "二、動作-單次取像", "三、動作-連續取像", "四、動作-儲存影像", "五、動作-閒置", "六、動作-離開", "CH1_Open", "CH2_Open", "CH3_Open", "CH4_Open", "CH1_Close", "CH2_Close", "CH3_Close", "CH4_Close", "Action1", "Action2", "Action3", "Action4", "Action5", "Action6", "Action7", "Action8", "Action9", "Action10", "Action11", "Action12", "Action13", "Action14", "Action15"]
        n189 = for {
          tunnel: w416 -> [w420]
          tunnel: [w419] -> w415
          tunnel: w417 -> [w418] mode=indexing
          n190 = Enqueue Element(queue=w420, element=w418) -> (queue out=w419:refnum<queue>)  [unwired: 2 in, 2 out]
        }
      }
      frame "Action14" {
        w423 = T3[] [enum."五、動作-閒置"] items=["一、動作-初始化", "二、動作-單次取像", "三、動作-連續取像", "四、動作-儲存影像", "五、動作-閒置", "六、動作-離開", "CH1_Open", "CH2_Open", "CH3_Open", "CH4_Open", "CH1_Close", "CH2_Close", "CH3_Close", "CH4_Close", "Action1", "Action2", "Action3", "Action4", "Action5", "Action6", "Action7", "Action8", "Action9", "Action10", "Action11", "Action12", "Action13", "Action14", "Action15"]
        n191 = for {
          tunnel: w422 -> [w426]
          tunnel: [w425] -> w421
          tunnel: w423 -> [w424] mode=indexing
          n192 = Enqueue Element(queue=w426, element=w424) -> (queue out=w425:refnum<queue>)  [unwired: 2 in, 2 out]
        }
      }
      frame "Action15" {
        w429 = T3[] [enum."五、動作-閒置"] items=["一、動作-初始化", "二、動作-單次取像", "三、動作-連續取像", "四、動作-儲存影像", "五、動作-閒置", "六、動作-離開", "CH1_Open", "CH2_Open", "CH3_Open", "CH4_Open", "CH1_Close", "CH2_Close", "CH3_Close", "CH4_Close", "Action1", "Action2", "Action3", "Action4", "Action5", "Action6", "Action7", "Action8", "Action9", "Action10", "Action11", "Action12", "Action13", "Action14", "Action15"]
        n193 = for {
          tunnel: w428 -> [w432]
          tunnel: [w431] -> w427
          tunnel: w429 -> [w430] mode=indexing
          n194 = Enqueue Element(queue=w432, element=w430) -> (queue out=w431:refnum<queue>)  [unwired: 2 in, 2 out]
        }
      }
    }
    "error out 2" <- w153
  }
  n195 = Index Array(array=w4, index=0) -> ()  [unwired: 1 out]
  n196 = Release Queue(queue=w11) -> ()  [unwired: 2 in, 3 out]
